vi "SVPWMTimingabcSGL_src.vi"(0 "A":sgl, 1 "max":sgl=0.9999695 caption="max voltage", 2 "Period":u32, 5 "B":sgl, 7 "C":sgl) -> (4 "U_Timing":T1, 6 "V_Timing":T1, 8 "W_timing":T1, 15 "Sector":u8)   [LabVIEW 2015]
uses:
  ON_OFF_timing.ctl
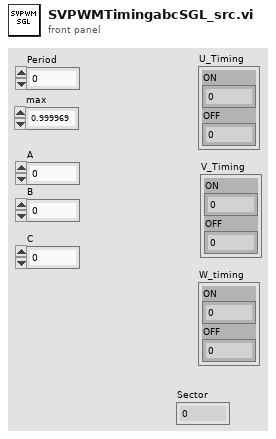
[diagram p1: front panel]
types:
  T1 = typedef "ON_OFF_timing.ctl" = cluster{"ON":u32, "OFF":u32}
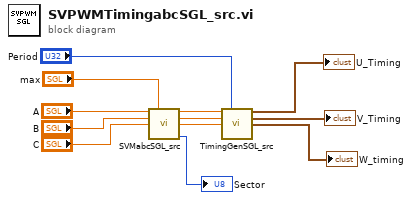
[diagram p0: block diagram]
diagram:
  n1 = call "SVMabcSGL_src.vi"("A"="A", "max"="max", "B"="B", "C"="C") -> ("Upercent"=w12:sgl, "Vpercent"=w11:sgl, "Wpercent"=w10:sgl, "Sector"=→"Sector":u8)  [unwired: 8 in]
  n2 = call "TimingGenSGL_src.vi"("Upercent"=w12, "Period"="Period", "Vpercent"=w11, "Wpercent"=w10) -> ("U_Timing"=→"U_Timing":T1, "V_Timing"=→"V_Timing":T1, "W_timing"=→"W_timing":T1)  [unwired: 9 in]
